vi "NMR10F.vi"() -> ()   [LabVIEW 2013]
uses:
  <vilib>/Analysis/NI_AALBase.lvlib
panel:
  out "RF OK":bool=TRUE
  out "Peak area (V-MHz)":sgl=0.26806173 format="%.3f"
  in  "Gauss Fit":bool
  out "NMR Graph + Fit":cluster{cluster{dbl, "Numeric":dbl}[]}[](graph)
  in  "Amp of Q curve":dbl=16.5 format="%_3f"
  in  "Subtract Q curve":bool=TRUE
  in  "Adjust Tune":bool=TRUE
  out "IF Offset":dbl(graph)=3.131691772460936
  out "Pedestal Difference":dbl(graph)=0.04542741927075716
  out "# Good Spectra":i32=99
  in  "Quality cuts":bool=TRUE
  out "Pedestal OK":bool=TRUE
  out "Sweep #":i32=2
  out "1st Sweep":bool
  out "ADC volts OK":bool=TRUE
  out "Peak Height Distribution":cluster{"Y":dbl[], "Y":dbl[]}[](graph)=[{"Y"=[0.2355519843953429, 0.23617339654540798, 0.2367948086954731, 0.2374162208455382, 0.2380376329956033, 0.2386590451456684, 0.23928045729573352, 0.2399018694457986, 0.24052328159586372, 0.2411446937459288, 0.24176610589599393, 0.24238751804605904, 0.24300893019612413, 0.24363034234618924, 0.24425175449625433, 0.24487316664631945, 0.24549457879638456, 0.24611599094644965, 0.24673740309651476, 0.24735881524657988, 0.24798022739664496, 0.24860163954671008, 0.24922305169677517, 0.24984446384684028, 0.2504658759969054, 0.2510872881469705, 0.25170870029703557, 0.2523301124471007, 0.2529515245971658, 0.2535729367472309, 0.25419434889729603, 0.25481576104736114, 0.2554371731974262, 0.2560585853474913, 0.25667999749755643, 0.25730140964762155, 0.25792282179768666, 0.2585442339477517, 0.25916564609781684, 0.25978705824788195, 0.26040847039794707, 0.2610298825480122, 0.26165129469807724, 0.26227270684814236, 0.26289411899820747, 0.2635155311482726, 0.2641369432983377, 0.26475835544840276, 0.2653797675984679, 0.266001179748533, 0.2666225918985981, 0.2672440040486632, 0.26786541619872833, 0.2684868283487934, 0.2691082404988585, 0.2697296526489236, 0.27035106479898874, 0.27097247694905385, 0.2715938890991189, 0.272215301249184, 0.27283671339924914, 0.27345812554931426, 0.27407953769937937, 0.27470094984944443, 0.27532236199950955, 0.27594377414957466, 0.2765651862996398, 0.2771865984497049, 0.27780801059976995, 0.27842942274983506, 0.2790508348999002, 0.2796722470499653, 0.2802936592000304, 0.2809150713500955, 0.2815364835001606, 0.2821578956502257, 0.2827793078002908, 0.28340071995035593, 0.28402213210042104, 0.2846435442504861, 0.2852649564005512, 0.28588636855061633, 0.28650778070068145, 0.28712919285074656, 0.2877506050008116, 0.28837201715087674, 0.28899342930094185, 0.28961484145100697, 0.2902362536010721, 0.29085766575113714, 0.29147907790120225, 0.29210049005126737, 0.2927219022013325, 0.2933433143513976, 0.2939647265014627, 0.2945861386515278, 0.2952075508015929, 0.295828962951658, 0.2964503751017231, 0.29707178725178823], "Y"=[1.0, 0.0, 0.0, 0.0, 0.0, 0.0, 0.0, 0.0, 0.0, 0.0, 0.0, 1.0, 0.0, 0.0, 1.0, 0.0, 0.0, 0.0, 0.0, 0.0, 0.0, 0.0, 1.0, 1.0, 0.0, 1.0, 1.0, 2.0, 0.0, 1.0, 3.0, 1.0, 1.0, 0.0, 3.0, 2.0, 2.0, 2.0, 3.0, 2.0, 0.0, 4.0, 1.0, 1.0, 4.0, 3.0, 3.0, 2.0, 4.0, 0.0, 4.0, 2.0, 3.0, 1.0, 1.0, 2.0, 4.0, 4.0, 3.0, 0.0, 3.0, 4.0, 2.0, 2.0, 1.0, 2.0, 0.0, 1.0, 0.0, 0.0, 1.0, 2.0, 0.0, 0.0, 1.0, 1.0, 1.0, 0.0, 0.0, 1.0, 0.0, 0.0, 0.0, 0.0, 0.0, 1.0, 0.0, 0.0, 0.0, 0.0, 0.0, 0.0, 0.0, 0.0, 0.0, 0.0, 0.0, 0.0, 0.0, 1.0]}]
  in  "# of Sweeps":i32=100
  out "Std Dev (V)":dbl=0.009965193633611454 format="%_2g"
  out "Peak mean (V)":dbl=0.2655884316981644 format="%_4g"
  out "Peak Height":dbl(graph)=0.26806171289062286
  in  "Raw Data":bool
  in  "Tank RF ON":bool=TRUE
  in  "IF Atten (dB)":i8 min=0 max=35 step=5
  in  "IFoffset (V)":dbl=3.131691772460936 min=0.0 max=3000.0 step=0.001 format="%.3f"
  in  "Tune  (V)":dbl=1.5059999999999982 min=0.0 max=5.0 step=0.001 format="%.3f"
  in  "Hi / Lo Gain":bool
  out "Voltage Array":sgl[](array[numeric])=[0.39486083, 0.39415282, 0.37740478, 0.36463624, 0.35776368, 0.33198243, 0.3107544, 0.32425538, 0.2953125, 0.27941895, 0.2874756, 0.2617798, 0.2520508, 0.24379882, 0.24141845, 0.22194824, 0.19313964, 0.1977295, 0.19276123, 0.17390136, 0.17283936, 0.16755371, 0.14387207, 0.12849121, 0.12796631, 0.13111572, 0.1216919, 0.10755615, 0.08287354, 0.06949463, 0.07113037, 0.062060546, 0.036108397, 0.032678224, 0.013000488, 0.0095825195, 0.01607666, 0.0040771486, 0.005566406, -0.01229248, 0.0024536133, -0.0022338866, -0.017175293, -0.029064942, -0.02878418, -0.05206299, -0.04116211, -0.05924072, -0.060913086, -0.07078858, -0.06147461, -0.0708252, -0.09482422, -0.09287109, -0.08811035, -0.10527344, -0.10979004, -0.09885254, -0.10852051, -0.12213135, -0.12347412, -0.13558349, -0.13809815, -0.1430664, -0.16062012, -0.16202393, -0.16688232, -0.1687622, -0.1630371, -0.17376709, -0.19066162, -0.17672119, -0.19134521, -0.19102784, -0.20743409, -0.1963379, -0.19866943, -0.20877686, -0.2253662, -0.21699218, -0.22194824, -0.22015381, -0.22921142, -0.21680908, -0.21575928, -0.23323974, -0.21798095, -0.22463378, -0.23702392, -0.21989746, -0.22541504, -0.20744629, -0.202063, -0.19719239, -0.18527833, -0.18197021, -0.13729247, -0.11975098, -0.061206054, -0.022375489, 0.010229493, 0.036230467, -0.003857422, -0.054382324, -0.0927124, -0.12541504, -0.1385376, -0.15421143, -0.16003418, -0.15662841, -0.19451904, -0.18380126, -0.19353028, -0.19848633, -0.19445801, -0.21176758, -0.20693359, -0.19925538, -0.19172363, -0.18999024, -0.19869384, -0.18461914, -0.19050293, -0.18470459, -0.18983154, -0.1901001, -0.20270996, -0.18931885, -0.18898925, -0.16983643, -0.17060547, -0.16373292, -0.16271973, -0.16048583, -0.1584961, -0.1397461, -0.14522704, -0.1364624, -0.13929443, -0.13120118, -0.11820068, -0.09746094, -0.105810545, -0.11616211, -0.11202393, -0.0831543, -0.08693848, -0.07366943, -0.076123044, -0.06868897, -0.05710449, -0.052990723, -0.0430542, -0.017224122, -0.010522461, -0.02224121, 0.0063842773, 0.0071655274, 0.009472656, 0.024536133, 0.02734375, 0.017590333, 0.036035158, 0.04018555, 0.06090088, 0.066381834, 0.084106445, 0.078625485, 0.09157715, 0.09299316, 0.107104495, 0.11695556, 0.118334964, 0.1282959, 0.134375, 0.17685547, 0.15549317, 0.17213134, 0.19041748, 0.2119873, 0.21591797, 0.22495118, 0.23574218, 0.23773193, 0.2640869, 0.2647583, 0.27943116, 0.28809816, 0.30527344, 0.32390136, 0.32923585, 0.334021, 0.34277344, 0.3604126, 0.37745363, 0.3977661, 0.40411377, 0.4104004, 0.42994386, 0.43033448, 0.4552002] format="%.4f"
  in  "Invert Polarity":bool=TRUE
  out "Pedestal Diff (V)":sgl=0.04542742 format="%.3f"
  out "Peak amp (V)":sgl=0.26806173 format="%.3f"
  in  "Save Data to File":bool
  in  "RF Level (dBm)":dbl=-2.0000000000000004 min=-10.0 max=1.0 step=0.1 format="%.2f"
  out "SMT error out":errorcluster
  out "Sample RMS (V)":dbl=0.014719094355728133 format="%.4f"
  in  "# Sample/step":i32=100 min=1 max=1000 step=100
  in  "ADC Rate (Hz)":i32=10000 min=1 max=20000 step=1000
  in  "ADC Range":i32(ring)=1 items=["+- 10 V"=1, "+- 2.5 V"=3]
  in  "Step Width (MHz)":dbl=0.002 min=0.0 max=1000.0 step=0.0005 format="%.4f"
  in  "Freq Span (MHz)":dbl=0.4 min=0.0 max=3000.0 step=0.1 format="%.3f"
  in  "Center Freq (MHz)":dbl=224.79 min=0.005 max=6000.0 step=0.1 format="%.3f"
  in  "Sweep Mode":u16(ring)=3 items=["Off", "Single", "Auto", "Step"]
  in  "GPIB Addr (28)":refnum<visa-resource-name>="GPIB0::28::INSTR"
  # "E1039 Prototype NMR Control Panel"
  # "Settings"
  # "D\nA\nC"
  # "R\nF\n\nG\ne\nn\ne\nr\na\nt\no\nr"
  # "A\nD\nC"
  # "D\na\nt\na"
  # "I\n/\nO"
  # "Results"
  # "A\nv\ne\nr\na\ng\ne"
  # "S\nw\ne\ne\np"
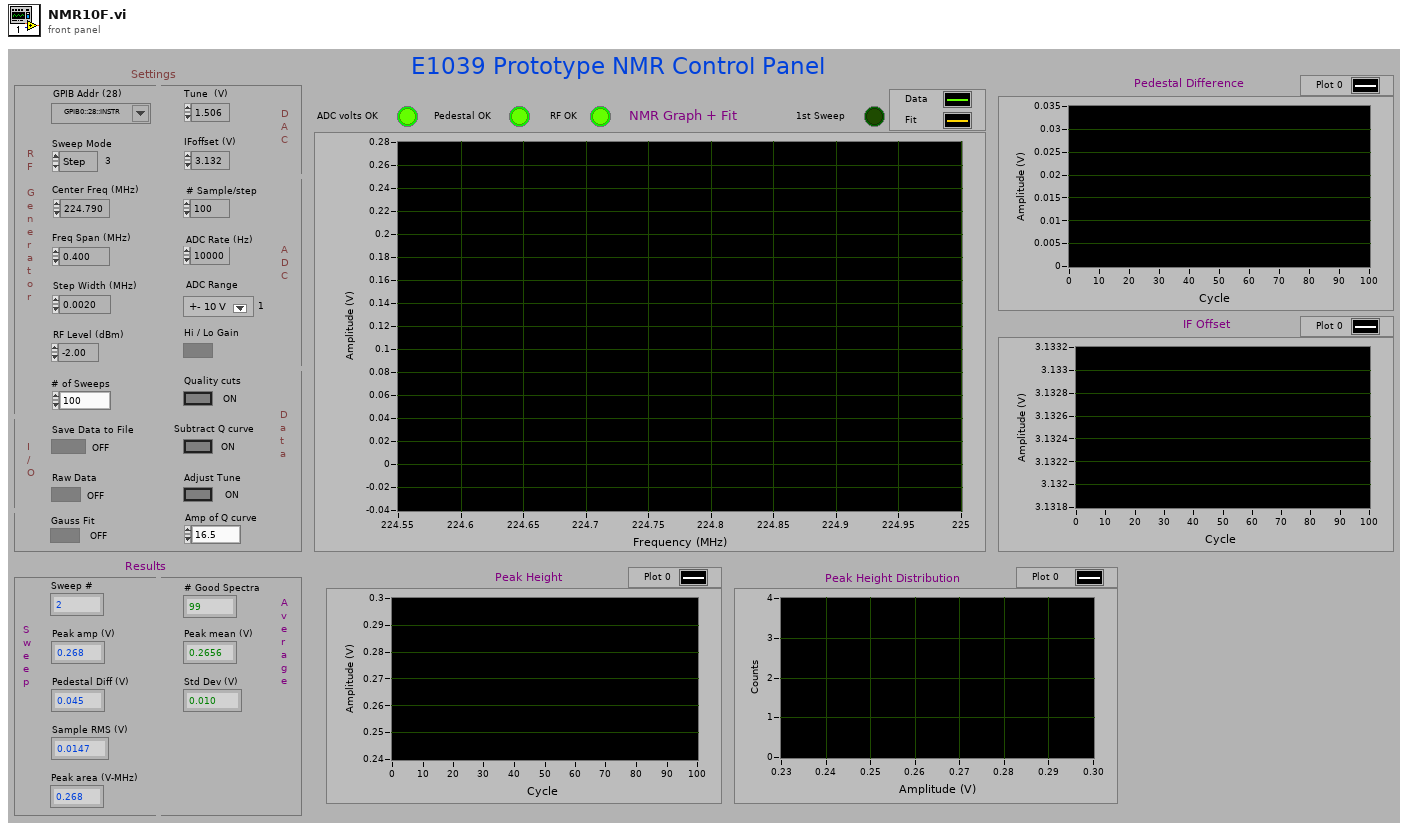
[diagram p1: front panel]
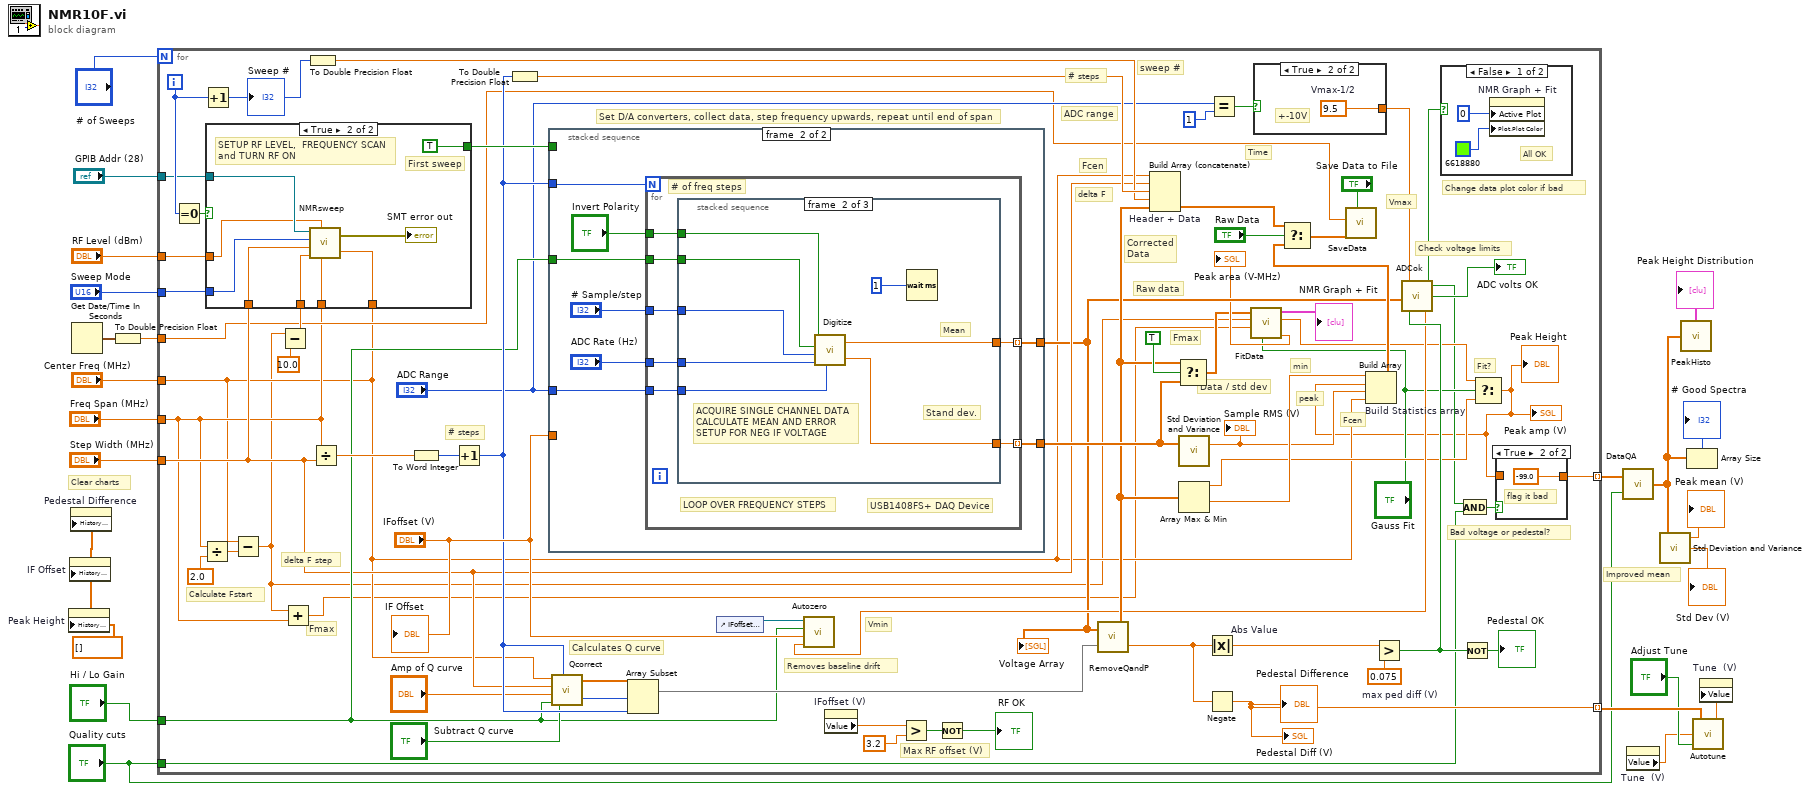
[diagram p0: block diagram]
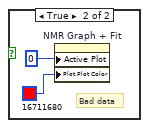
[diagram p2: hidden frame]
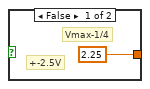
[diagram p3: hidden frame]
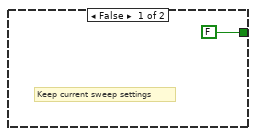
[diagram p5: hidden frame]
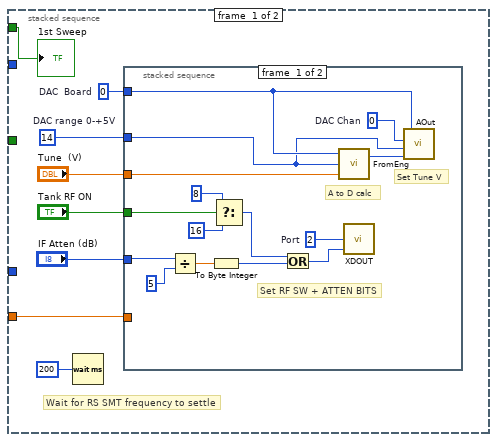
[diagram p6: hidden frame]
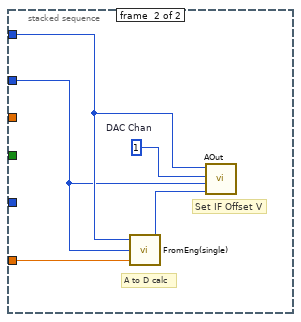
[diagram p7: hidden frame]
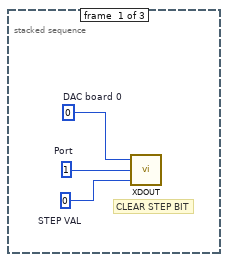
[diagram p8: hidden frame]
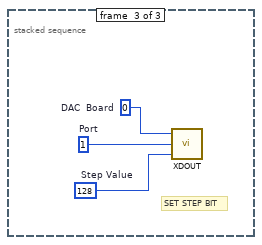
[diagram p9: hidden frame]
diagram:
  w6 = dbl[] []
  # "Clear charts"
  # "Improved mean"
  n1 = property on="Peak Height" class="WFChart (strict)"("History Data"=w6) -> ()  [unwired: 2 in, 2 out]
  n2 = property on="IF Offset" class="WFChart (strict)"("History Data"=w6) -> ()  [unwired: 2 in, 2 out]
  n3 = property on="Pedestal Difference" class="WFChart (strict)"("History Data"=w6) -> ()  [unwired: 2 in, 2 out]
  n4 = Get Date/Time In Seconds() -> (seconds since 1Jan1904=w2:timestamp)
  n5 = To Double Precision Float(number=w2) -> (double precision float=w1:dbl)
  n6 = for {
    N: "# of Sweeps" -> [_]
    tunnel: [w73] -> w18 mode=indexing
    tunnel: "Quality cuts" -> [w45]
    tunnel: [w54] -> w15 mode=indexing
    tunnel: "Center Freq (MHz)" -> [w32]
    tunnel: "Freq Span (MHz)" -> [w38]
    tunnel: "Step Width (MHz)" -> [w44]
    tunnel: "Sweep Mode" -> [w58]
    tunnel: "Hi / Lo Gain" -> [w57]
    tunnel: "GPIB Addr (28)" -> [w56]
    tunnel: "RF Level (dBm)" -> [w55]
    tunnel: w1 -> [w39]
    i -> [w71]
    w74 = 0.075  # max ped diff (V)
    # "Vmax"
    # "Change data plot color if bad"
    # "Max RF offset (V)"
    # "Fmax"
    # "Fit?"
    # "Fmax"
    # "Time"
    # "Vmin"
    # "min"
    # "peak"
    # "Raw data"
    # "Corrected\nData"
    # "Fcen"
    # "delta F"
    # "# steps"
    # "ADC range"
    # "sweep #"
    # "Fcen"
    # "Set D/A converters, collect data, step frequency upwards, repeat until end of span"
    # "Calculates Q curve"
    # "Removes baseline drift"
    # "Bad voltage or pedestal?"
    # "Check voltage limits"
    # "Data / std dev"
    # "# steps"
    # "Calculate Fstart"
    # "delta F step"
    n7 = Equal To 0?(x=w71) -> (x = 0?=w76:bool)
    n8 = Divide(x=w38, y=sgl 2.0) -> (x/y=w88:dbl)
    n9 = Increment(x=w71) -> (x+1=w61:i32)
    "Sweep #" <- w61
    n10 = Subtract(x=w32, y=w88) -> (x-y=w27:dbl)
    n11 = Subtract(x=w27, y=10.0) -> (x-y=w86:dbl)
    n12 = case shown="True" w76 {
      tunnel: w86 -> [_ w108]
      tunnel: w44 -> [_ w106]
      tunnel: w32 -> [_ w105]
      tunnel: w38 -> [_ w107]
      tunnel: [FALSE TRUE] -> w75
      tunnel: w58 -> [_ w102]
      tunnel: w56 -> [_ w101]
      tunnel: w55 -> [_ w100]
      frame False {
        # "Keep current sweep settings"
      }
      frame True {
        # "First sweep"
        # "SETUP RF LEVEL,  FREQUENCY SCAN\nand TURN RF ON"
        n13 = call "NMRsweep.vi"("Center Freq (MHz)"=w105, "Freq Span (MHz)"=w107, "RF Level (dBm)"=w100, "Foffset (MHz)"=w108, "Step Width (MHz)"=w106, "Sweep Mode"=w102, "GPIB Addr (28)"=w101) -> ("error out"=→"SMT error out":errorcluster)
      }
    }
    n14 = Add(x=w27, y=w38) -> (x+y=w26:dbl)
    n15 = To Double Precision Float(number=w61) -> (double precision float=w62:dbl)
    n16 = Divide(x=w38, y=w44) -> (x/y=w90:dbl)
    n17 = To Word Integer(number=w90) -> (16bit integer=w87:i16)
    n18 = Increment(x=w87) -> (x+1=w65:i16)
    n19 = To Double Precision Float(number=w65) -> (double precision float=w64:dbl)
    n20 = stacked-sequence {
      tunnel: [_ w144] -> w79
      tunnel: [_ w143] -> w42
      tunnel: w65 -> [_ w142]
      tunnel: "IFoffset (V)" -> [w110 _]
      tunnel: w57 -> [_ w141]
      tunnel: w75 -> [w109 _]
      tunnel: "ADC Range" -> [_ w140]
      frame #0 {
        w114 = 14  # DAC range 0-+5V
        w115 = 0  # DAC  Board
        # "Wait for RS SMT frequency to settle"
        n21 = Wait (ms)(milliseconds to wait=200) -> ()  [unwired: 1 out]
        n22 = stacked-sequence {
          tunnel: w115 -> [w122 w134]
          tunnel: w114 -> [w121 w133]
          tunnel: "Tune  (V)" -> [w120 _]
          tunnel: "Tank RF ON" -> [w118 _]
          tunnel: "IF Atten (dB)" -> [w117 _]
          tunnel: w110 -> [_ w132]
          frame #0 {
            w124 = 2  # Port
            w131 = 0  # DAC Chan
            # "A to D calc"
            # "Set RF SW + ATTEN BITS"
            # "Set Tune V"
            n23 = Divide(x=w117, y=5) -> (x/y=w129:dbl)
            n24 = To Byte Integer(number=w129) -> (8bit integer=w126:i8)
            n25 = Select(t=8, s=w118, f=16) -> (s? t:f=w125:i32)
            n26 = Or(x=w125, y=w126) -> (x .or. y?=w123:i32)
            n27 = call-poly "FromEng.VI"("Eng Units"=w120, "Range"=w121, "BoardNum (0)"=w122) -> ("DA Data"=w119:u16)  [unwired: 1 out]
            n28 = call "XDOUT.VI"(2:w123, "PortNum"=w124) -> ()  [unwired: 3 in]
            n29 = call "AOut.VI"("DataValue"=w119, "Range"=w121, "Channel"=w131, "BoardNum"=w122) -> ()  [unwired: 1 out]
          }
          frame #1 {
            w136 = 1  # DAC Chan
            # "A to D calc"
            # "Set IF Offset V"
            n30 = call "FromEng(single).VI"("Eng Units"=w132, "Range"=w133, "BoardNum (0)"=w134) -> ("DA Data"=w135:u16)  [unwired: 1 out]
            n31 = call "AOut.VI"("DataValue"=w135, "Range"=w133, "Channel"=w136, "BoardNum"=w134) -> ()  [unwired: 1 out]
          }
        }
        "1st Sweep" <- w109
      }
      frame #1 {
        n32 = for {
          N: w142 -> [_]
          tunnel: [w151] -> w143 mode=indexing
          tunnel: [w150] -> w144 mode=indexing
          tunnel: w141 -> [w149]
          tunnel: w140 -> [w148]
          tunnel: "ADC Rate (Hz)" -> [w147]
          tunnel: "# Sample/step" -> [w146]
          tunnel: "Invert Polarity" -> [w145]
          # "# of freq steps"
          # "USB1408FS+ DAQ Device"
          # "LOOP OVER FREQUENCY STEPS"
          n33 = stacked-sequence {
            tunnel: [_ w161 _] -> w151
            tunnel: [_ w160 _] -> w150
            tunnel: w149 -> [_ w159 _]
            tunnel: w148 -> [_ w158 _]
            tunnel: w147 -> [_ w157 _]
            tunnel: w146 -> [_ w156 _]
            tunnel: w145 -> [_ w155 _]
            frame #0 {
              w152 = 0  # DAC board 0
              w153 = 0  # STEP VAL
              w154 = 1  # Port
              # "CLEAR STEP BIT"
              n34 = call "XDOUT.VI"(2:w153, "PortNum"=w154, "BoardNum"=w152) -> ()  [unwired: 2 in]
            }
            frame #1 {
              # "Stand dev."
              # "Mean"
              # "ACQUIRE SINGLE CHANNEL DATA\nCALCULATE MEAN AND ERROR\nSETUP FOR NEG IF VOLTAGE"
              n35 = call "Digitize.vi"("Invert Polarity"=w155, "IF or Log"=w159, "# Sample/step"=w156, "ADC Rate (Hz)"=w157, "ADC Range"=w158) -> ("mean"=w161:dbl, "standard deviation"=w160:dbl)
              n36 = Wait (ms)(milliseconds to wait=1) -> ()  [unwired: 1 out]
            }
            frame #2 {
              w163 = 128  # Step Value
              w165 = 0  # DAC  Board
              w164 = 1  # Port
              # "SET STEP BIT"
              n37 = call "XDOUT.VI"(2:w163, "PortNum"=w164, "BoardNum"=w165) -> ()  [unwired: 2 in]
            }
          }
        }
      }
    }
    "Voltage Array" <- w42
    n38 = call "Qcorrect.vi"("Subtract Q curve"="Subtract Q curve", "Nstep"=w65, "IF or Log"=w57, "Amp of Q curve"="Amp of Q curve", "Step Width (MHz)"=w44, "Center Freq (MHz)"=w32) -> ("Start"=w81:i32, "Array"=w82:dbl[])
    n39 = Array Subset "Array Subset"(array=w82, index=w81, length=w65) -> (w80:dbl[])
    n40 = control-ref of="IFoffset (V)"() -> (w48:refnum<vi>)
    n41 = property on="IFoffset (V)" class="DigNum (strict)"() -> ("Value"=w36:dbl)  [unwired: 2 in, 2 out]
    n42 = Greater?(x=w36, y=3.2) -> (0:w34:bool)
    n43 = Not(x=w34) -> (.not. x?=→"RF OK":bool)
    n44 = call "RemoveQandP.vi"("Qcurve"=w80, "Raw data"=w42) -> ("Ped L-R"=w67:dbl, "Corrected data"=w63:dbl[])
    n45 = Build Array (concatenate) "Header + Data"(w32, w44, w64, w62, w63) -> (w66:dbl[])
    n46 = Select(t=w63, s=TRUE, f=w79) -> (s? t:f=w28:dbl[])
    n47 = call <vilib>:"Std Deviation and Variance.vi"("X"=w79) -> ("mean"=w43:dbl)  [unwired: 1 in, 2 out]
    "Sample RMS (V)" <- w43
    n48 = Array Max & Min(array=w63) -> (max value=w37:dbl, min value=w78:dbl)  [unwired: 2 out]
    n49 = Absolute Value "Abs Value"(x=w67) -> (abs(x)=w69:dbl)
    n50 = Negate(x=w67) -> (-x=w54:dbl)
    "Pedestal Diff (V)" <- w54
    "Pedestal Difference" <- w54
    n51 = Equal?(x="ADC Range", y=1) -> (x = y?=w52:bool)
    n52 = call "FitData.vi"("Fit?"="Gauss Fit", "Fmax"=w26, "Fmin"=w27, "Yarray"=w28) -> ("Peak Area (V-MHz)"=→"Peak area (V-MHz)":dbl, "Amplitude (V)"=w30:dbl, "NMR Graph + Fit"=→"NMR Graph + Fit":cluster{cluster{dbl, "Numeric":dbl}[]}[])  [unwired: 2 out]
    n53 = case shown="True" w52 {
      tunnel: [2.25 w96] -> w49
      frame False {
        # "Vmax-1/4"
        # "+-2.5V"
      }
      frame True {
        w96 = 9.5  # Vmax-1/2
        # "+-10V"
      }
    }
    n54 = Greater?(x=w69, y=w74) -> (0:w53:bool)
    n55 = call "ADCok.vi"("PedOK"=w53, "Array"=w42, "Vmax-1/2"=w49) -> ("Vmin"=w47:dbl, "ADC voltages OK"=→"ADC volts OK":bool, "Allok"=w24:bool)
    n56 = call "Autozero.vi"("Vmin (V)"=w47, "IFoffset (V)"="IFoffset (V)", "IF or Log"=w57, "reference"=w48) -> ()
    n57 = case shown="False" w24 {
      frame False {
        # "All OK"
        n58 = property on="NMR Graph + Fit" class="XYGraph (strict)"("Active Plot"=0, "Plot.Plot Color"=u32 6618880) -> ()  [unwired: 2 in, 2 out]
      }
      frame True {
        # "Bad data"
        n59 = property on="NMR Graph + Fit" class="XYGraph (strict)"("Active Plot"=0, "Plot.Plot Color"=u32 16711680) -> ()  [unwired: 2 in, 2 out]
      }
    }
    n60 = And(x=w24, y=w45) -> (x .and. y?=w70:bool)
    n61 = Not(x=w53) -> (.not. x?=→"Pedestal OK":bool)
    n62 = Select(t=w30, s="Gauss Fit", f=w37) -> (s? t:f=w23:dbl)
    "Peak amp (V)" <- w23
    "Peak Height" <- w23
    n63 = Build Array "Build Statistics array"(w78, w23, w43, w32) -> (w85:dbl[])
    n64 = Select(t=w66, s="Raw Data", f=w85) -> (s? t:f=w40:dbl[])
    n65 = call "SaveData.vi"("Array"=w40, "Save Data to File"="Save Data to File", "Ext time (sec)"=w39) -> ()  [unwired: 1 out]
    n66 = case shown="True" w70 {
      tunnel: [w97 -99.0] -> w73
      tunnel: w23 -> [w97 _]
      frame False {
        # "Data OK"
      }
      frame True {
        # "flag it bad"
      }
    }
    "IF Offset" <- "IFoffset (V)"
  }
  n67 = call "DataQA.vi"("Quality cuts"="Quality cuts", "Data In"=w18) -> ("Data Out"=w17:dbl[])
  n68 = property on="Tune  (V)" class="DigNum (strict)"() -> ("Value"=w5:dbl)  [unwired: 2 in, 2 out]
  n69 = call <vilib>:"Std Deviation and Variance.vi"("X"=w17) -> ("mean"=→"Peak mean (V)":dbl, "standard deviation"=→"Std Dev (V)":dbl)  [unwired: 1 in, 1 out]
  n70 = call "PeakHisto.vi"("Data Out"=w17) -> ("XY Graph"=→"Peak Height Distribution":cluster{"Y":dbl[], "Y":dbl[]}[])
  n71 = Array Size(array=w17) -> (size(s)=→"# Good Spectra":i32)
  n72 = call "Autotune.vi"("Adjust Tune"="Adjust Tune", "Tune Vin"=w5, "Pedestal Diff"=w15) -> ("Tune Vout"=w4:dbl)
  n73 = property on="Tune  (V)" class="DigNum (strict)"("Value"=w4) -> ()  [unwired: 2 in, 2 out]
